vi "Instrument Add.vi"(8 "error in (no error)":errorcluster, 10 "Instrument Record":T2, 11 "Connection Refnum":T1) -> (0 "error out":errorcluster, 2 "New Instrument Record":T2, 3 "Connection Refnum":T1)   [LabVIEW 2011]
uses:
  Instrument Record.ctl
  Summitek EXT/ODBC/SQL Controls/Connection Refnum.ctl
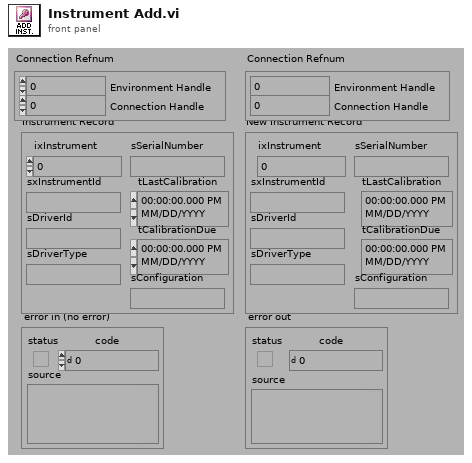
[diagram p1: front panel]
types:
  T1 = typedef "Connection Refnum.ctl" = cluster{"Environment Handle":i32, "Connection Handle":i32}
  T2 = typedef "Instrument Record.ctl" = cluster{"ixInstrument":i32, "sxInstrumentId":string, "sDriverId":string, "sDriverType":string, "sSerialNumber":string, "tLastCalibration":timestamp, "tCalibrationDue":timestamp, "sConfiguration":string}
  T3 = typedef "Statement Refnum.ctl" = cluster{"Statement Handle":i32, "Parameter Number":u16}
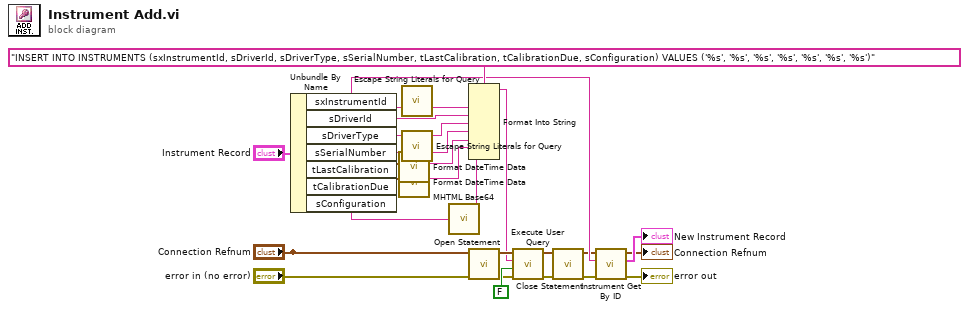
[diagram p0: block diagram]
diagram:
  n1 = Unbundle By Name("Instrument Record") -> ("sxInstrumentId"=w3:string, "sDriverId"=w12:string, "sDriverType"=w11:string, "sSerialNumber"=w6:string, "tLastCalibration"=w10:timestamp, "tCalibrationDue"=w7:timestamp, "sConfiguration"=w16:string)
  n2 = call "Format DateTime Data.vi"("Timestamp in"=w10) -> ("UTC DB String out"=w9:string)  [unwired: 10 out]
  n3 = call "Format DateTime Data.vi"("Timestamp in"=w7) -> ("UTC DB String out"=w8:string)  [unwired: 10 out]
  n4 = call "Escape String Literals for Query.vi"("String"=w3) -> ("escaped String"=w5:string)  [unwired: 1 in, 13 out]
  n5 = call "Escape String Literals for Query.vi"("String"=w6) -> ("escaped String"=w4:string)  [unwired: 1 in, 13 out]
  n6 = call "MHTML Base64.vi"("Binary String"=w16) -> ("String (Base64)"=w15:string)  [unwired: 14 out]
  n7 = Format Into String(format string="INSERT INTO INSTRUMENTS (sxInstrumentId, sDriverId, sDriverType, sSerialNumber, tLastCalibration, tCalibrationDue, sConfiguration) VALUES ('%s', '%s', '%s', '%s', '%s', '%s', '%s')" ("User Query"), w5, w12, w11, w4, w9, w8, w15) -> (resulting string=w18:string)  [unwired: 2 in, 1 out]
  n8 = call "Open Statement.vi"("error in (no error)"="error in (no error)", "Connection Refnum"="Connection Refnum") -> ("error out"=w21:errorcluster, "Statement Refnum"=w20:T3)  [unwired: 4 out]
  n9 = call "Execute User Query.vi"("error in (no error)"=w21, "Return Data? (f)"=FALSE, "User Query"=w18, "Statement Refnum"=w20) -> ("error out"=w23:errorcluster, "Statement Refnum"=w24:T3)  [unwired: 2 out]
  n10 = call "Close Statement.vi"("error in (no error)"=w23, "Statement Refnum"=w24) -> ("error out"=w17:errorcluster)  [unwired: 5 out]
  n11 = call "Instrument Get By ID.vi"("error in (no error)"=w17, "sxInstrumentId (\"\")"=w3, "Connection Refnum"="Connection Refnum") -> ("error out"=→"error out":errorcluster, "Instrument Record"=→"New Instrument Record":T2, "Connection Refnum"=→"Connection Refnum":T1)  [unwired: 6 out]
